vi "ACT_LabVIEW_2p1_Team072.vi"() -> ()   [LabVIEW 2016]
uses:
  <vilib>/express/express arith-compare/Formula/XNode/ExpressFormulaBlockNode.xnode
panel:
  in  "New Unit In":string(combo)
  out "New Unit Out":string
  out "Mass,":dbl
  in  "Mass, kg":dbl
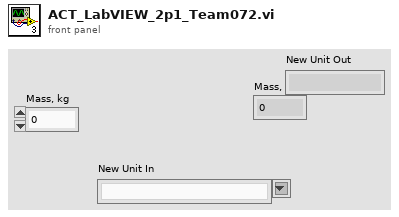
[diagram p1: front panel]
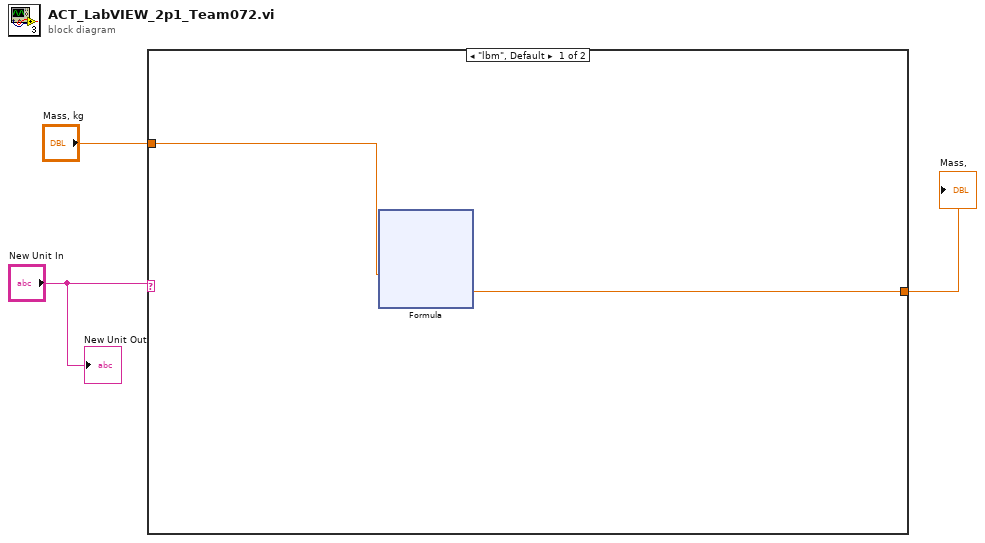
[diagram p0: block diagram]
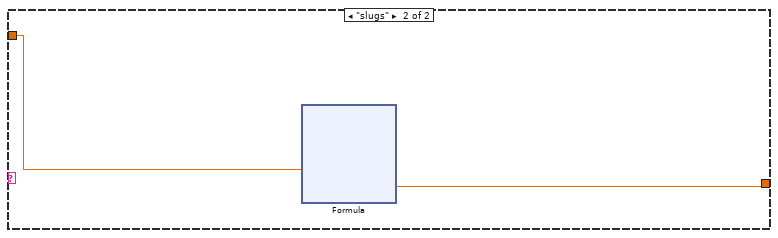
[diagram p2: hidden frame]
diagram:
  n1 = case shown="\"lbm\", Default" "New Unit In" {
    tunnel: "Mass, kg" -> [w5 w15]
    tunnel: [w4 w14] -> w2
    frame "lbm", Default {
      n2 = xnode "Formula"("m"=w5) -> ("Result"=w4:dbl)  [unwired: 1 in, 1 out]
    }
    frame "slugs" {
      n3 = xnode "Formula"("m"=w15) -> ("Result"=w14:dbl)  [unwired: 1 in, 1 out]
    }
  }
  "Mass," <- w2
  "New Unit Out" <- "New Unit In"
